vi "Write Cluster Size.vi"(5 "Cluster Size":T1, 9 "Cluster in":refnum<class "Cluster.lvclass">) -> (3 "Cluster out":refnum<class "Cluster.lvclass">)   [LabVIEW 2014, in "Raspberry Pi Compatible Compiler for LabVIEW.lvlib" / "Cluster.lvclass"]
uses:
  Cluster.lvclass
  <vilib>/Utility/miscctls.llb/LVBoundsTypeDef.ctl
  Cluster.lvclass/Cluster.ctl
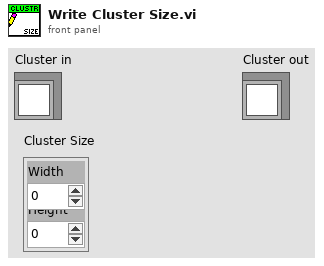
[diagram p1: front panel]
types:
  T1 = typedef "LVBoundsTypeDef.ctl" = cluster{"Width":u32, "Height":u32}
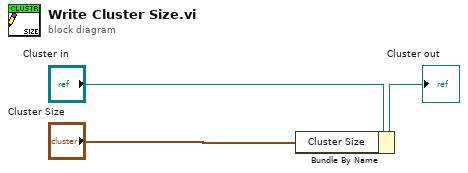
[diagram p0: block diagram]
diagram:
  n1 = Bundle By Name(cluster="Cluster in", "Cluster Size"="Cluster Size") -> (→"Cluster out":refnum<class "Cluster.lvclass">)
